vi "Basic Example.vi"() -> ()   [LabVIEW 2020, in "Current Value Table(Rebuild).lvlib"]
doc: "This VI demonstrates how to use the CVT."
uses:
  Current Value Table(Rebuild).lvlib
  Type Defs/Data Types.ctl
  Type Defs/Tag Grouping set.ctl
  Type Defs/File Format.ctl
  Type Defs/Single Tag.ctl
  DataTypes/Double_Write.vi
  DataTypes/Single_Read.vi
  DataTypes/Double_Static Read.vi
  DataTypes/I64_Read.vi
panel:
  in  "Tag 4":sgl
  in  "Tag 3":i64
  out "Tag 1":dbl
  in  "stop":bool
  out "error out":errorcluster
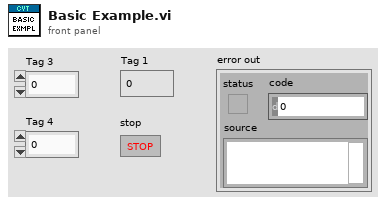
[diagram p1: front panel]
types:
  T1 = typedef "Current Value Table(Rebuild).lvlib/File Format.ctl" = cluster{"Tags":T2[], "Group Listings":T4[]}
  T2 = typedef "Current Value Table(Rebuild).lvlib/Single Tag.ctl" = cluster{"Data Type":T3, "Name":string, "Value":string, "Description":string}
  T3 = typedef "Current Value Table(Rebuild).lvlib/Data Types.ctl" = enum16{"Double", "Single", "I64", "I32", "I16", "I8", "U64", "U32", "U16", "U8", "String", "Boolean", "Array of U8", "Array of U16", "Array of U32", "Array of U64", "Array of I64", "Array of I32", "Array of I16", "Array of I8", "Array of Double", "Array of Single", "Array of Boolean", "Array of String"}
  T4 = typedef "Current Value Table(Rebuild).lvlib/Tag Grouping set.ctl" = cluster{"Group":string, "Tag Names":string[]}
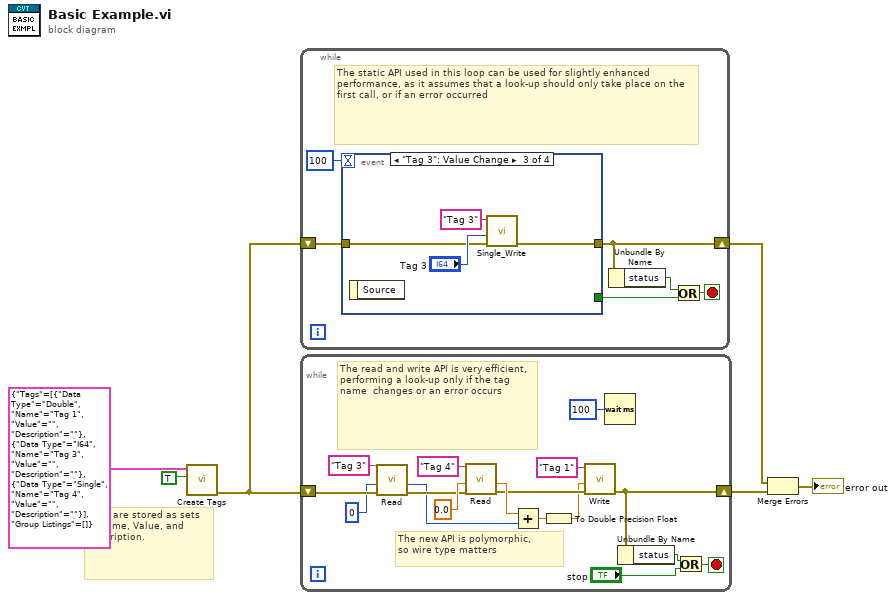
[diagram p0: block diagram]
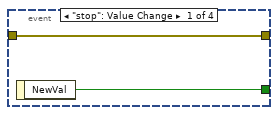
[diagram p2: hidden frame]
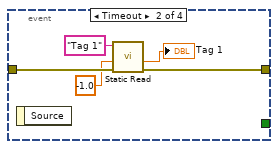
[diagram p3: hidden frame]
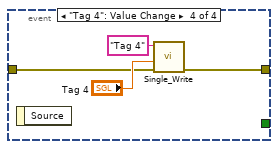
[diagram p4: hidden frame]
diagram:
  # "Tags are stored as sets of Name, Value, and Description."
  n1 = call "Create Tags.vi"("Clear Table? (F)"=TRUE ("Clear Engine?"), "CVT Tags to Create"=T1 {"Tags"=[{"Data Type"=enum."Double", "Name"="Tag 1", "Value"="", "Description"=""}, {"Data Type"=enum."I64", "Name"="Tag 3", "Value"="", "Description"=""}, {"Data Type"=enum."Single", "Name"="Tag 4", "Value"="", "Description"=""}], "Group Listings"=[]} ("CVT File Data")) -> ("error out"=w1:errorcluster)  [unwired: 9 in]
  n2 = while {
    shift-right: [w8] -> w3
    shift-left: w1 -> [w9]
    stop <- w11 stop-if-true
    # "The static API used in this loop can be used for slightly enhanced performance, as it assumes that a look-up should only take place on the first call, or if an error occurred"
    n3 = event shown="[2] \"Tag 3\": Value Change" {
      selector: _ -> [_ _ _ _]
      dyn-events: _ -> [_ _ _ _]
      timeout: 100 -> [_ _ _ _]
      tunnel: [w14 _ _ _] -> w12
      tunnel: [w13 w16 w23 w27] -> w8
      tunnel: w9 -> [w13 w17 w20 w24]
      event "stop": Value Change {
        n4 = event-data() -> ("NewVal"=w14:bool)  [unwired: 1 in]
      }
      event Timeout {
        n5 = event-data() -> ()  [unwired: 1 in, 1 out]
        n6 = call-poly "Static Read.vi"("error in (no error)"=w17, "Default"=-1.0, "Tag Name"="Tag 1") -> ("error out"=w16:errorcluster, "Value"=→"Tag 1":dbl)  [unwired: 7 in]
      }
      event "Tag 3": Value Change {
        n7 = event-data() -> ()  [unwired: 1 in, 1 out]
        n8 = call "Single_Write.vi"("error in (no error)"=w20, "Value"="Tag 3", "Tag Name"="Tag 3") -> ("error out"=w23:errorcluster)  [unwired: 8 in]
      }
      event "Tag 4": Value Change {
        n9 = event-data() -> ()  [unwired: 1 in, 1 out]
        n10 = call "Single_Write.vi"("error in (no error)"=w24, "Value"="Tag 4", "Tag Name"="Tag 4") -> ("error out"=w27:errorcluster)  [unwired: 8 in]
      }
    }
    n11 = Unbundle By Name(w8) -> ("status"=w7:bool)
    n12 = Or(x=w7, y=w12) -> (x .or. y?=w11:bool)
  }
  n13 = while {
    shift-right: [w29] -> w4
    shift-left: w1 -> [w44]
    stop <- w31 stop-if-true
    # "The read and write API is very efficient, performing a look-up only if the tag name  changes or an error occurs"
    # "The new API is polymorphic,\nso wire type matters"
    n14 = call-poly "Read.vi"("error in (no error)"=w44, "Default"=i64 0, "Tag Name"="Tag 3") -> ("error out"=w39:errorcluster, "Value"=w37:i64)  [unwired: 7 in]
    n15 = call-poly "Read.vi"("error in (no error)"=w39, "Default"=sgl 0.0, "Tag Name"="Tag 4") -> ("error out"=w36:errorcluster, "Value"=w38:sgl)  [unwired: 7 in]
    n16 = Add(x=w38, y=w37) -> (x+y=w35:sgl)
    n17 = To Double Precision Float(number=w35) -> (double precision float=w34:dbl)
    n18 = call-poly "Write.vi"("error in (no error)"=w36, "Value"=w34, "Tag Name"="Tag 1") -> ("error out"=w29:errorcluster)  [unwired: 8 in]
    n19 = Wait (ms)(milliseconds to wait=u32 100) -> ()  [unwired: 1 out]
    n20 = Unbundle By Name(w29) -> ("status"=w28:bool)
    n21 = Or(x=w28, y="stop") -> (x .or. y?=w31:bool)
  }
  n22 = Merge Errors(w3, w4) -> (→"error out":errorcluster)
